vi "Encode Fixed Header.vi"(8 "error in (no error)":errorcluster, 11 "Fixed Header":T1) -> (0 "error out":errorcluster, 3 "String":string)   [LabVIEW 2017, in "WebSocket.lvclass"]
uses:
  WebSocket.lvclass
  private/Fixed Header.ctl
  private/OpCode.ctl
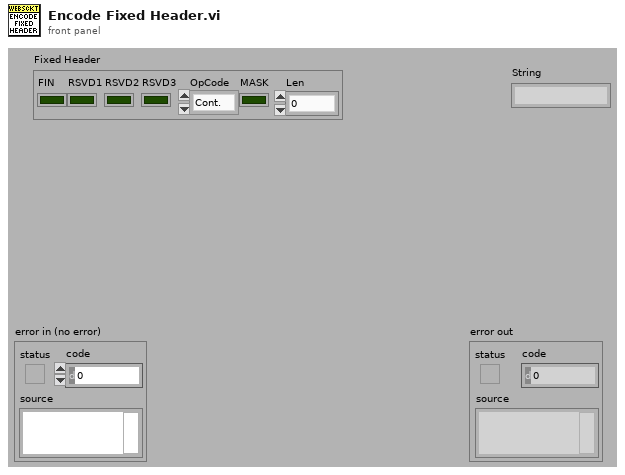
[diagram p1: front panel]
types:
  T1 = typedef "WebSocket.lvclass/Fixed Header.ctl" = cluster{"FIN":bool, "RSVD1":bool, "RSVD2":bool, "RSVD3":bool, "OpCode":T2, "MASK":bool, "Len":u8}
  T2 = typedef "WebSocket.lvclass/OpCode.ctl" = enum16{"Cont.", "Text", "Binary", "NonCtl3", "NonCtl4", "NonCtl5", "NonCtl6", "NonCtl7", "Close", "Ping", "Pong", "Rsvd11", "Rsvd12", "Rsvd13", "Rsvd14", "Rsvd15"}
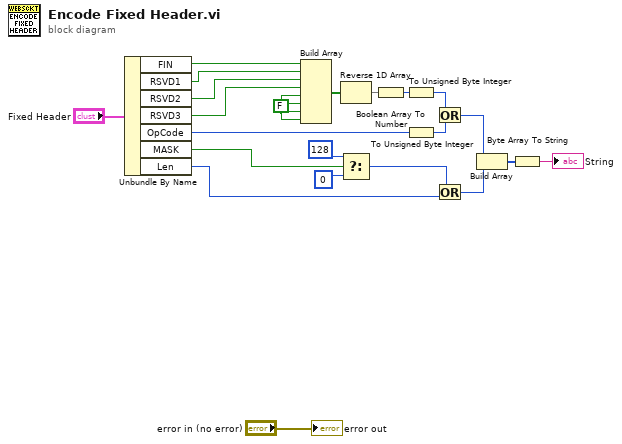
[diagram p0: block diagram]
diagram:
  w16 = FALSE
  n1 = Unbundle By Name("Fixed Header") -> ("FIN"=w20:bool, "RSVD1"=w19:bool, "RSVD2"=w18:bool, "RSVD3"=w17:bool, "OpCode"=w13:T2, "MASK"=w6:bool, "Len"=w9:u8)
  n2 = Build Array(w20, w19, w18, w17, w16, w16, w16, w16) -> (w15:bool[])
  n3 = Reverse 1D Array(array=w15) -> (reversed array=w14:bool[])
  n4 = Select(t=u8 128 ("Len"), s=w6, f=u8 0 ("Len")) -> (s? t:f=w8:u8)
  n5 = Boolean Array To Number(Boolean array=w14) -> (number=w12:u32)
  n6 = To Unsigned Byte Integer(number=w12) -> (unsigned 8bit integer=w11:u8)
  n7 = To Unsigned Byte Integer(number=w13) -> (unsigned 8bit integer=w10:u8)
  n8 = Or(x=w11, y=w10) -> (x .or. y?=w3:u8)
  n9 = Or(x=w8, y=w9) -> (x .or. y?=w4:u8)
  n10 = Build Array(w3, w4) -> (w2:u8[])
  n11 = Byte Array To String(unsigned byte array=w2) -> (string=→"String":string)
  "error out" <- "error in (no error)"
